vi "Derivative of graph.vi"() -> ()   [LabVIEW 2016]
uses:
  <vilib>/Analysis/NI_AALPro.lvlib
panel:
  out "XY Graph 2":cluster{dbl[], dbl[]}[](graph)
  in  "Section selection":enum32{"Curve Array section", "Curve section"}(tab)
  in  "Sec of curve array ?":bool=TRUE
  out "Data array size(s)":i32=6
  in  "length 3":i32=1
  in  "Starting 3":i32
  in  "Plot.Line Style for tangent curve":u8=1
  out "Each tangent curve":cluster{dbl[], dbl[]}(graph)
  in  "X Array for plotting tangent curves":dbl[](array[numeric])=[0.0]
  out "XY Graph":cluster{dbl[], dbl[]}[](graph)
  out "Curve Zero point":cluster{"X":dbl, "Y":dbl, "slope":dbl}={"X"=-8.080417881800293e-06, "Y"=-1.1123375641542113e-11, "slope"=1.7801191832269458e-09}
  out "Curve last":cluster{"X":dbl, "Y":dbl, "slope":dbl}={"X"=0.3798387285276693, "Y"=3.107099170942364e-09, "slope"=3.198705006979033e-08}
  out "Curve first":cluster{"X":dbl, "Y":dbl, "slope":dbl}={"X"=-0.3635330617914448, "Y"=-1.8462257979443692e-09, "slope"=1.561085352493134e-08}
  out "Closest value":dbl=-8.080417881800293e-06
  out "Max":dbl=3.865032587499246e-08
  out "Min":dbl=3.353872771127181e-10
  out "Half maximum":dbl=1.949285657605259e-08
  out "size(s) of X array":i32=4999
  in  "A vs B":cluster{dbl[], dbl[]}[](graph)=[{array[4999 elements], array[4999 elements]}, {array[4999 elements], array[4999 elements]}, {array[4999 elements], array[4999 elements]}, {array[4999 elements], array[4999 elements]}, {array[4999 elements], array[4999 elements]}, {array[4999 elements], array[4999 elements]}]
  in  "dy/dx vs x":bool=TRUE
  in  "Numeric":dbl=100.0
  out "A vs B 3":cluster{dbl[], dbl[]}[](graph)
  # "Attention: When false, it plots dx/dy vs y"
  # "Choose range of curve array"
  # "Choose range of each curve"
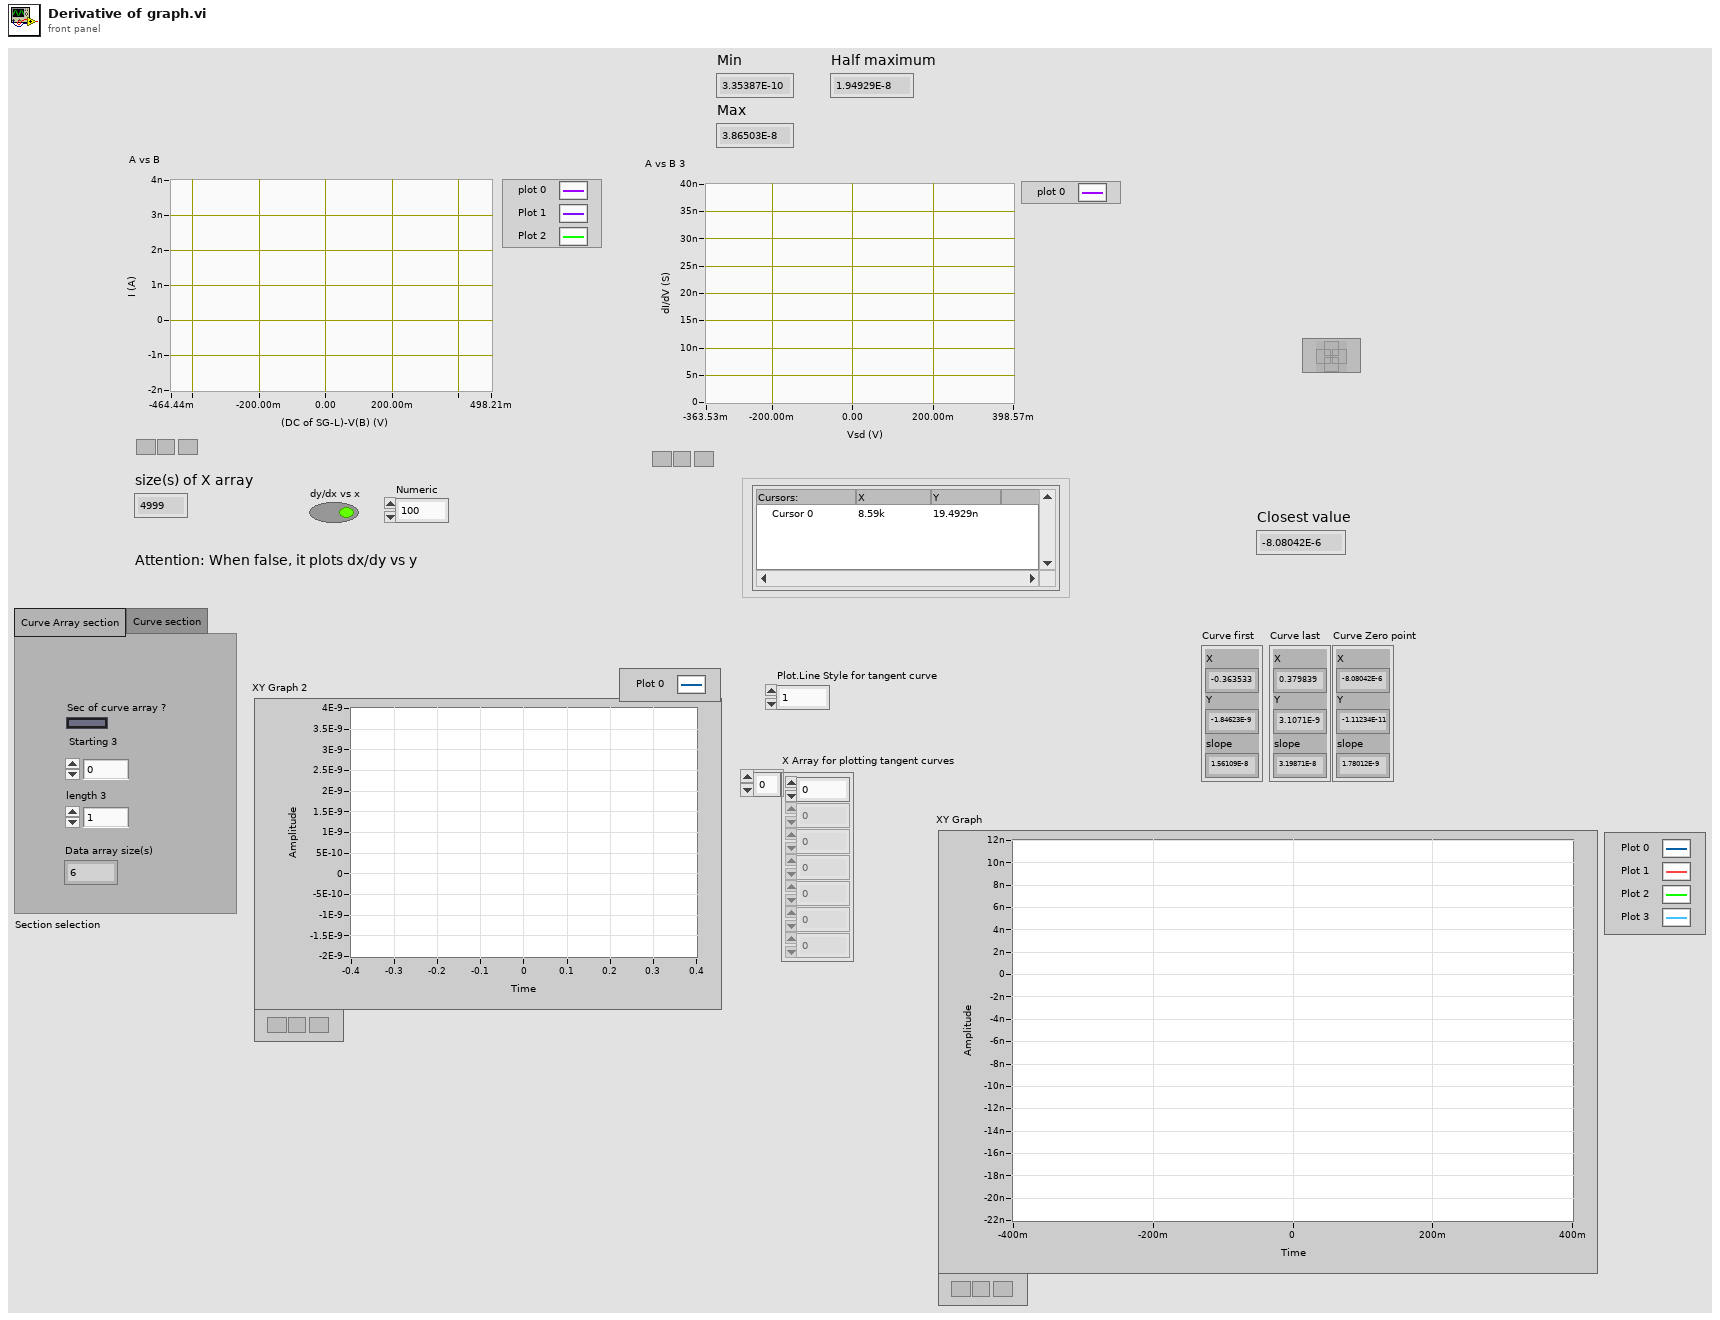
[diagram p1: front panel]
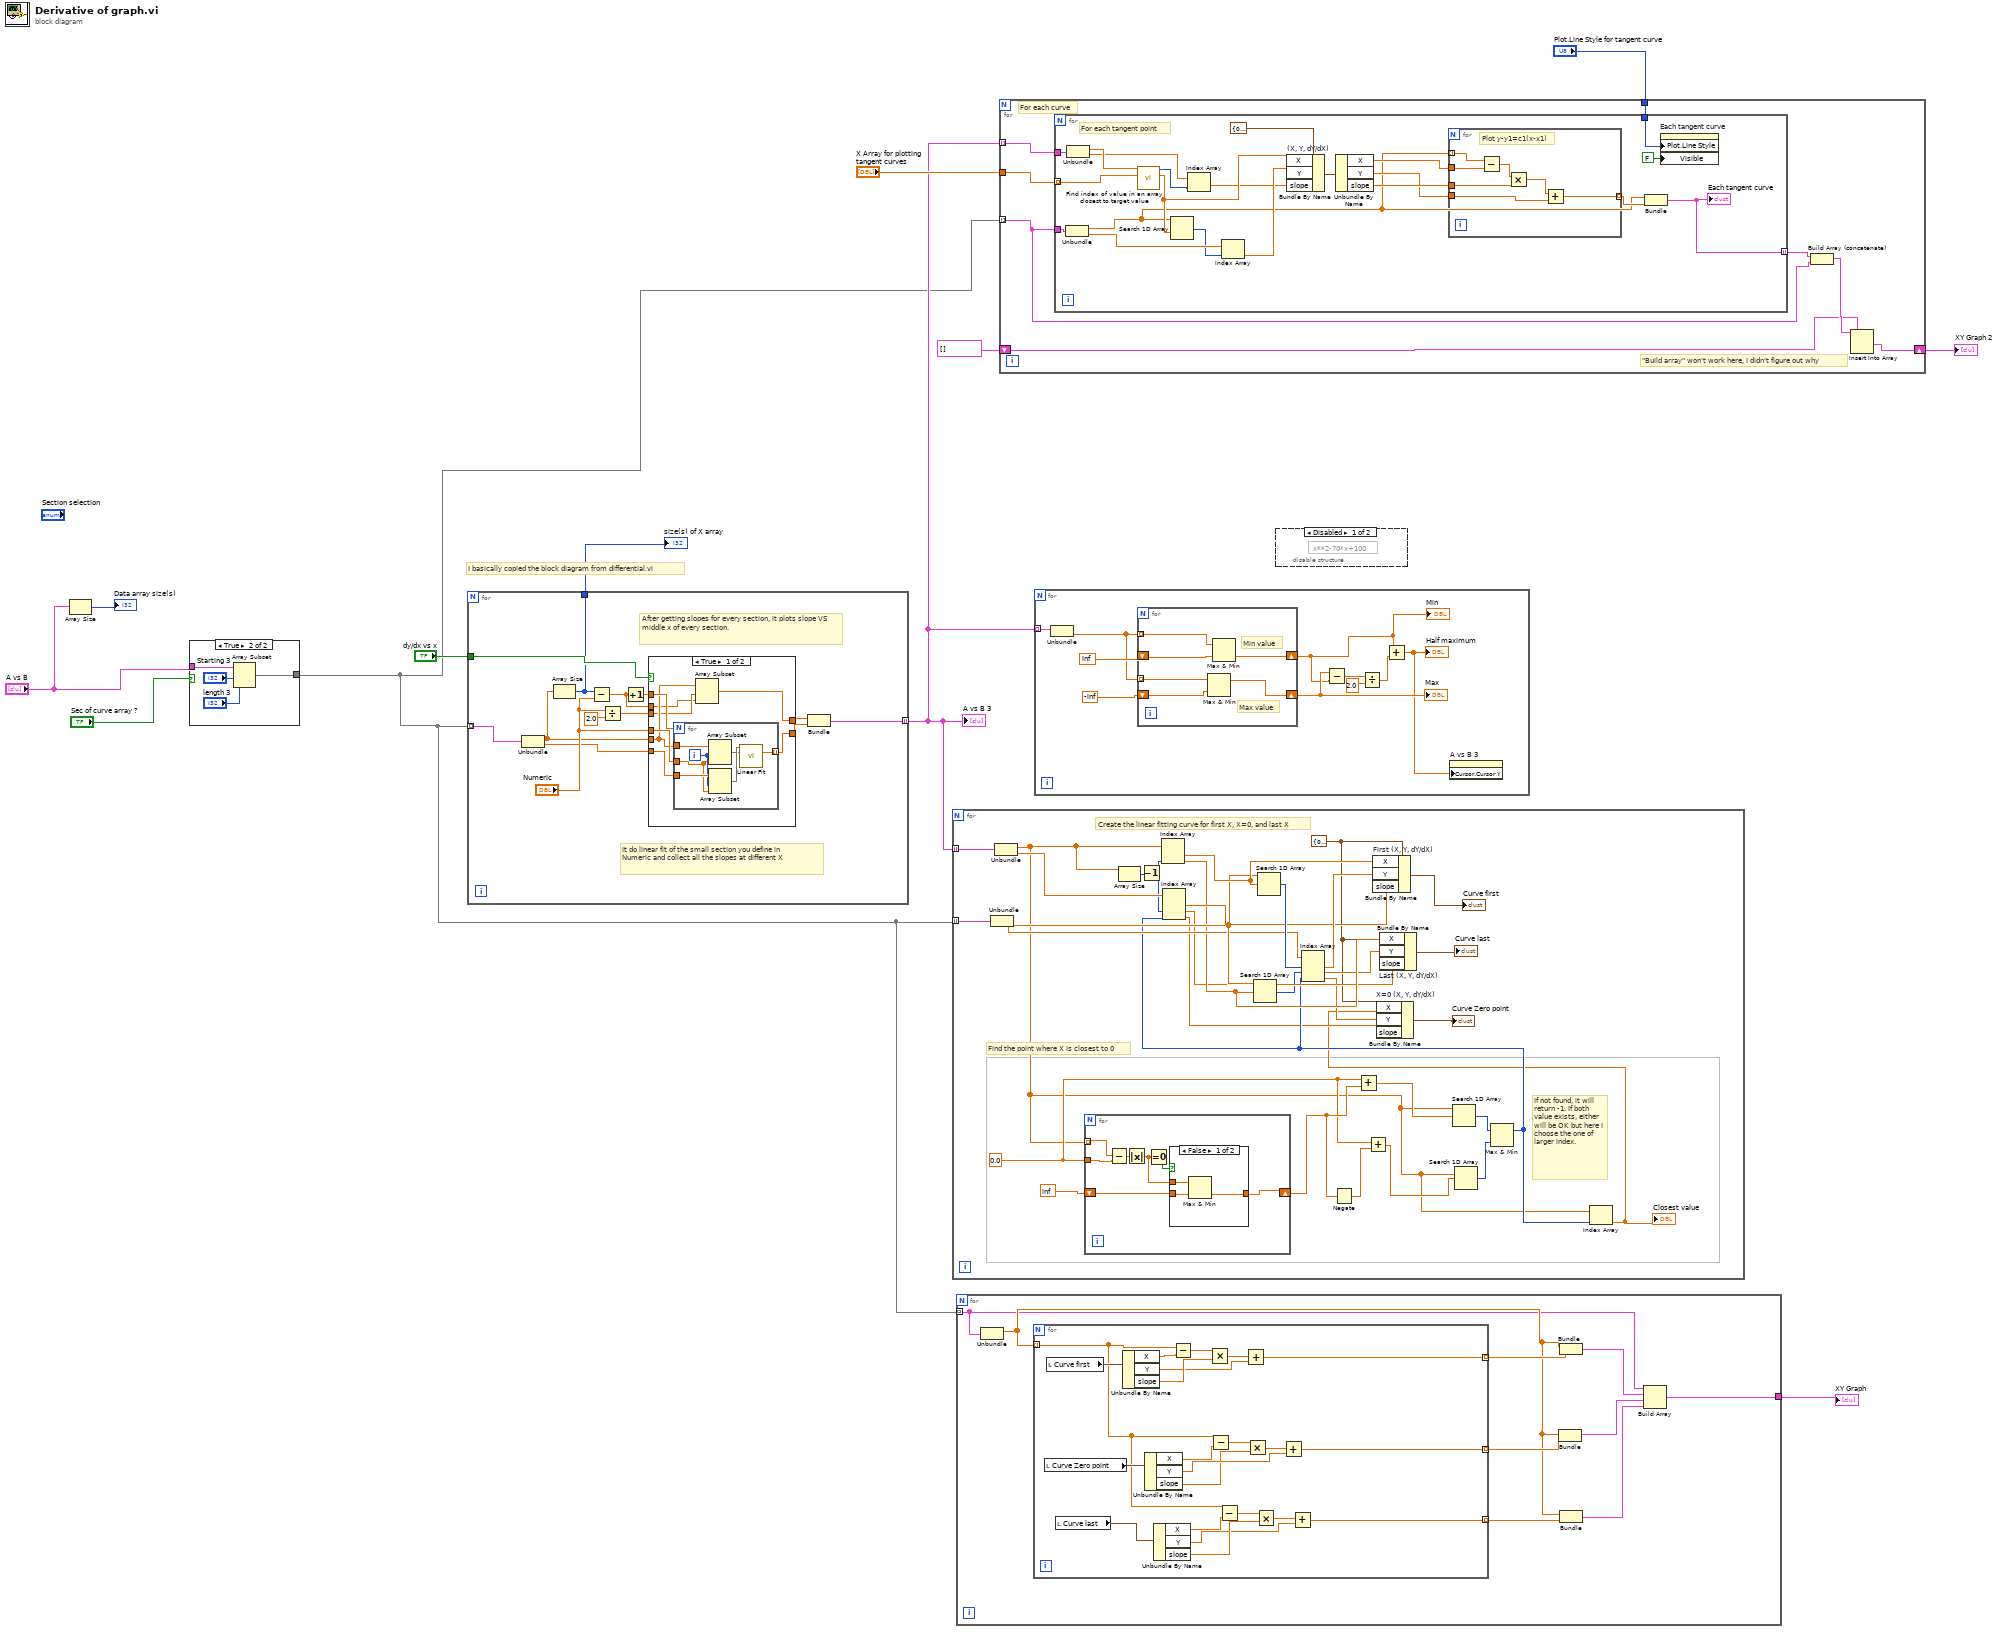
[diagram p0: block diagram]
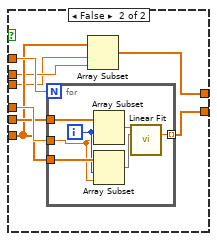
[diagram p5: hidden frame]
diagram:
  # "I basically copied the block diagram from differential.vi"
  n1 = Array Size(array="A vs B") -> (size(s)=→"Data array size(s)":i32)
  n2 = case shown="True" "Sec of curve array ?" {
    tunnel: "A vs B" -> [w13 w17]
    tunnel: [w13 w14] -> w5
    frame False {
    }
    frame True {
      n3 = Array Subset(array=w17, index="Starting 3", length="length 3") -> (w14:cluster{dbl[], dbl[]}[])
    }
  }
  n4 = for {
    tunnel: [w22] -> w8 mode=indexing
    tunnel: w5 -> [w21] mode=indexing
    tunnel: "dy/dx vs x" -> [w20]
    tunnel: [w19] -> w11
    # "After getting slopes for every section, it plots slope VS middle x of every section."
    # "It do linear fit of the small section you define in Numeric and collect all the slopes at different X"
    n5 = Unbundle(w21) -> (w18:dbl[], w26:dbl[])
    n6 = Array Size(array=w18) -> (size(s)=w19:i32)
    n7 = Subtract(x=w19, y="Numeric") -> (x-y=w24:dbl)
    n8 = Divide(x="Numeric", y=2.0) -> (x/y=w25:dbl)
    n9 = Increment(x=w24) -> (x+1=w30:dbl)
    n10 = case shown="True" w20 {
      tunnel: w30 -> [w38 w53]
      tunnel: "Numeric" -> [w37 w52]
      tunnel: [w36 w51] -> w27
      tunnel: w18 -> [w34 w50]
      tunnel: w26 -> [w35 w49]
      tunnel: w25 -> [w33 w47]
      tunnel: w24 -> [w32 w48]
      tunnel: [w31 w46] -> w23
      frame True {
        n11 = for {
          N: w38 -> [_]
          tunnel: w34 -> [w45]
          tunnel: w35 -> [w44]
          tunnel: w37 -> [w42]
          tunnel: [w41] -> w36 mode=indexing
          i -> [w43]
          n12 = Array Subset(array=w45, index=w43, length=w42) -> (w39:dbl[])
          n13 = Array Subset(array=w44, index=w43, length=w42) -> (w40:dbl[])
          n14 = call <vilib>:"Linear Fit.vi"("Y"=w40, "X"=w39) -> ("slope"=w41:dbl)  [unwired: 9 in, 4 out]
        }
        n15 = Array Subset(array=w34, index=w33, length=w32) -> (w31:dbl[])
      }
      frame False {
        n16 = for {
          N: w53 -> [_]
          tunnel: w50 -> [w60]
          tunnel: w49 -> [w59]
          tunnel: w52 -> [w57]
          tunnel: [w56] -> w51 mode=indexing
          i -> [w58]
          n17 = Array Subset(array=w60, index=w58, length=w57) -> (w55:dbl[])
          n18 = Array Subset(array=w59, index=w58, length=w57) -> (w54:dbl[])
          n19 = call <vilib>:"Linear Fit.vi"("Y"=w55, "X"=w54) -> ("slope"=w56:dbl)  [unwired: 9 in, 4 out]
        }
        n20 = Array Subset(array=w49, index=w47, length=w48) -> (w46:dbl[])
      }
    }
    n21 = Bundle(w23, w27) -> (w22:cluster{dbl[], dbl[]})  [unwired: 1 in]
  }
  "A vs B 3" <- w8
  "size(s) of X array" <- w11
  n22 = for {
    tunnel: w8 -> [w92] mode=indexing
    tunnel: w5 -> [w91] mode=indexing
    w62 = cluster{"X":dbl, "Y":dbl, "slope":dbl} {"X"=0.0, "Y"=0.0, "slope"=0.0} ("cluster")
    w71 = 0.0 ("x")
    # "Find the point where X is closest to 0"
    # "If not found, it will return -1. If both value exists, either will be OK but here I choose the one of larger index."
    # "Create the linear fitting curve for first X, X=0, and last X"
    n23 = Unbundle(w91) -> (w85:dbl[], w84:dbl[])
    n24 = Unbundle(w92) -> (w63:dbl[], w87:dbl[])
    n25 = for {
      tunnel: w63 -> [w95] mode=indexing
      shift-right: [w94] -> w75
      shift-left: inf -> [w99]
      tunnel: w71 -> [w93]
      n26 = Subtract(x=w95, y=w93) -> (x-y=w98:dbl)
      n27 = Absolute Value(x=w98) -> (abs(x)=w96:dbl)
      n28 = Equal To 0?(x=w96) -> (x = 0?=w97:bool)
      n29 = case shown="False" w97 {
        tunnel: w99 -> [w102 _]
        tunnel: [w101 w103] -> w94
        tunnel: w96 -> [w100 w103]
        frame False {
          n30 = Max & Min(x=w100, y=w102) -> (min(x,y)=w101:dbl)  [unwired: 1 out]
        }
        frame True {
        }
      }
    }
    n31 = Array Size(array=w63) -> (size(s)=w82:i32)
    n32 = Decrement(x=w82) -> (x-1=w61:i32)
    n33 = Index Array(array=w63, index #2=w61) -> (element #1=w89:dbl, element #2=w83:dbl)  [unwired: 1 in]
    n34 = Search 1D Array(1D array=w85, element=w83) -> (index of element=w79:i32)  [unwired: 1 in]
    n35 = Search 1D Array(1D array=w85, element=w89) -> (index of element=w90:i32)  [unwired: 1 in]
    n36 = Negate(x=w75) -> (-x=w73:dbl)
    n37 = Add(x=w71, y=w75) -> (x+y=w74:dbl)
    n38 = Add(x=w71, y=w73) -> (x+y=w72:dbl)
    n39 = Search 1D Array(1D array=w63, element=w74) -> (index of element=w77:i32)  [unwired: 1 in]
    n40 = Search 1D Array(1D array=w63, element=w72) -> (index of element=w76:i32)  [unwired: 1 in]
    n41 = Max & Min(x=w77, y=w76) -> (max(x,y)=w69:i32)  [unwired: 1 out]
    n42 = Index Array(array=w87, index #2=w61, index #3=w69) -> (element #1=w86:dbl, element #2=w81:dbl, element #3=w68:dbl)  [unwired: 1 in]
    n43 = Index Array(array=w84, index #1=w90, index #2=w79, index #3=w69) -> (element #1=w88:dbl, element #2=w80:dbl, element #3=w70:dbl)
    n44 = Bundle By Name "First (X, Y, dY/dX)"(cluster=w62, "X"=w89, "Y"=w88, "slope"=w86) -> (→"Curve first":cluster{"X":dbl, "Y":dbl, "slope":dbl})
    n45 = Bundle By Name "Last (X, Y, dY/dX)"(cluster=w62, "X"=w83, "Y"=w80, "slope"=w81) -> (→"Curve last":cluster{"X":dbl, "Y":dbl, "slope":dbl})
    n46 = Index Array(array=w63, index=w69) -> (element=w67:dbl)
    "Closest value" <- w67
    n47 = Bundle By Name "X=0 (X, Y, dY/dX)"(cluster=w62, "X"=w67, "Y"=w70, "slope"=w68) -> (→"Curve Zero point":cluster{"X":dbl, "Y":dbl, "slope":dbl})
  }
  n48 = for {
    tunnel: w5 -> [w104] mode=indexing
    tunnel: [w105] -> w10
    n49 = Unbundle(w104) -> (w109:dbl[])  [unwired: 1 out]
    n50 = for {
      tunnel: w109 -> [w117] mode=indexing
      tunnel: [w115] -> w112 mode=indexing
      tunnel: [w114] -> w111 mode=indexing
      tunnel: [w113] -> w110 mode=indexing
      n51 = local read "Curve Zero point"() -> (w126:cluster{"X":dbl, "Y":dbl, "slope":dbl})
      n52 = local read "Curve first"() -> (w134:cluster{"X":dbl, "Y":dbl, "slope":dbl})
      n53 = local read "Curve last"() -> (w116:cluster{"X":dbl, "Y":dbl, "slope":dbl})
      n54 = Unbundle By Name(w134) -> ("X"=w133:dbl, "Y"=w130:dbl, "slope"=w131:dbl)
      n55 = Unbundle By Name(w126) -> ("X"=w125:dbl, "Y"=w124:dbl, "slope"=w123:dbl)
      n56 = Unbundle By Name(w116) -> ("X"=w120:dbl, "Y"=w121:dbl, "slope"=w122:dbl)
      n57 = Subtract(x=w117, y=w133) -> (x-y=w132:dbl)
      n58 = Multiply(x=w132, y=w131) -> (x*y=w129:dbl)
      n59 = Subtract(x=w117, y=w125) -> (x-y=w127:dbl)
      n60 = Subtract(x=w117, y=w120) -> (x-y=w119:dbl)
      n61 = Add(x=w129, y=w130) -> (x+y=w115:dbl)
      n62 = Multiply(x=w127, y=w123) -> (x*y=w128:dbl)
      n63 = Multiply(x=w119, y=w122) -> (x*y=w118:dbl)
      n64 = Add(x=w128, y=w124) -> (x+y=w114:dbl)
      n65 = Add(x=w118, y=w121) -> (x+y=w113:dbl)
    }
    n66 = Bundle(w109, w111) -> (w107:cluster{dbl[], dbl[]})  [unwired: 1 in]
    n67 = Bundle(w109, w112) -> (w108:cluster{dbl[], dbl[]})  [unwired: 1 in]
    n68 = Bundle(w109, w110) -> (w106:cluster{dbl[], dbl[]})  [unwired: 1 in]
    n69 = Build Array(w104, w108, w107, w106) -> (w105:cluster{dbl[], dbl[]}[])
  }
  "XY Graph" <- w10
  n70 = for {
    tunnel: w8 -> [w142] mode=indexing
    tunnel: "X Array for plotting tangent curves" -> [w141]
    tunnel: w5 -> [w138] mode=indexing
    tunnel: "Plot.Line Style for tangent curve" -> [w140]
    shift-right: [w137] -> w2
    shift-left: cluster{dbl[], dbl[]}[] [] ("appended array") -> [w135]
    # "\"Build array\" won't work here, I didn't figure out why"
    # "For each curve"
    n71 = for {
      tunnel: w142 -> [w163]
      tunnel: w141 -> [w161] mode=indexing
      tunnel: w138 -> [w158]
      tunnel: w140 -> [w145]
      tunnel: [w143] -> w139 mode=indexing
      # "For each tangent point"
      n72 = Unbundle(w158) -> (w146:dbl[], w157:dbl[])
      n73 = Unbundle(w163) -> (w162:dbl[], w160:dbl[])
      n74 = call "Find index of value in an array closest to target value.vi"("Target value"=w161, "Array"=w162) -> ("Closest value"=w153:dbl, "Index of closest value"=w159:i32)  [unwired: 8 in]
      n75 = Search 1D Array(1D array=w146, element=w153) -> (index of element=w156:i32)  [unwired: 1 in]
      n76 = Index Array(array=w160, index=w159) -> (element=w152:dbl)
      n77 = Index Array(array=w157, index=w156) -> (element=w154:dbl)
      n78 = Bundle By Name "(X, Y, dY/dX)"(cluster=cluster{"X":dbl, "Y":dbl, "slope":dbl} {"X"=0.0, "Y"=0.0, "slope"=0.0}, "X"=w153, "Y"=w154, "slope"=w152) -> (w151:cluster{"X":dbl, "Y":dbl, "slope":dbl})
      n79 = Unbundle By Name(w151) -> ("X"=w150:dbl, "Y"=w148:dbl, "slope"=w149:dbl)
      n80 = for {
        tunnel: w146 -> [w170] mode=indexing
        tunnel: w150 -> [w169]
        tunnel: w149 -> [w167]
        tunnel: w148 -> [w166]
        tunnel: [w164] -> w147 mode=indexing
        # "Plot y-y1=c1(x-x1)"
        n81 = Subtract(x=w170, y=w169) -> (x-y=w168:dbl)
        n82 = Multiply(x=w168, y=w167) -> (x*y=w165:dbl)
        n83 = Add(x=w165, y=w166) -> (x+y=w164:dbl)
      }
      n84 = Bundle(w146, w147) -> (w143:cluster{dbl[], dbl[]})  [unwired: 1 in]
      "Each tangent curve" <- w143
      n85 = property on="Each tangent curve" class="XYGraph (strict)"("Plot.Line Style"=w145, "Visible"=FALSE) -> ()  [unwired: 2 in, 2 out]
    }
    n86 = Build Array (concatenate)(w139, w138) -> (w136:cluster{dbl[], dbl[]}[])
    n87 = Insert Into Array(array=w135, new element=w136) -> (w137:cluster{dbl[], dbl[]}[])  [unwired: 1 in]
  }
  "XY Graph 2" <- w2
  n88 = for {
    tunnel: w8 -> [w180] mode=indexing
    n89 = Unbundle(w180) -> (w178:dbl[])  [unwired: 1 out]
    n90 = for {
      tunnel: w178 -> [w185] mode=indexing
      shift-right: [w184] -> w173
      shift-left: inf -> [w186]
      tunnel: w178 -> [w183] mode=indexing
      shift-right: [w181] -> w176
      shift-left: -inf -> [w182]
      # "Max value"
      # "Min value"
      n91 = Max & Min(x=w183, y=w182) -> (max(x,y)=w181:dbl)  [unwired: 1 out]
      n92 = Max & Min(x=w185, y=w186) -> (min(x,y)=w184:dbl)  [unwired: 1 out]
    }
    "Min" <- w173
    "Max" <- w176
    n93 = Subtract(x=w176, y=w173) -> (x-y=w175:dbl)
    n94 = Divide(x=w175, y=2.0) -> (x/y=w172:dbl)
    n95 = Add(x=w173, y=w172) -> (x+y=w171:dbl)
    "Half maximum" <- w171
    n96 = property on="A vs B 3" class="XYGraph (strict)"("Cursor.Cursor Y"=w171) -> ()  [unwired: 2 in, 2 out]
  }
  n97 = disable-structure shown="Disabled" {
    frame Disabled {
      n98 = expression code="x**2-70*x+100"() -> ()  [unwired: 1 in, 1 out]
    }
    frame Enabled {
    }
  }
